vi "qCOV.vi"(0 "System no.":i32=1 min=1 max=4 step=1, 2 "ID to query":string[](array[string]), 3 "All IDs?":bool, 5 "error in":errorcluster) -> (14 "OL Velocity":dbl[](array[numeric]) format="%.6f", 19 "error out":errorcluster)   [LabVIEW 2020]
doc: "Returns current open loop velocity for specified IDs.\n\nE-870: Only one ID to query per command allowed."
panel:
  # "Returns current open loop velocity for specified IDs."
  # "Query"
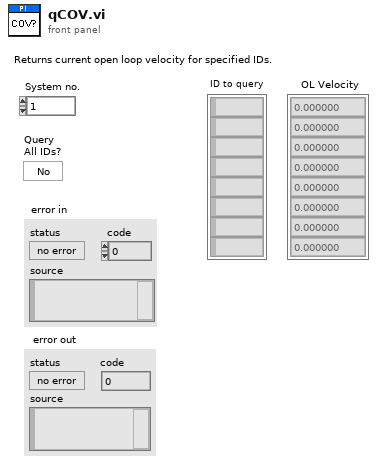
[diagram p1: front panel]
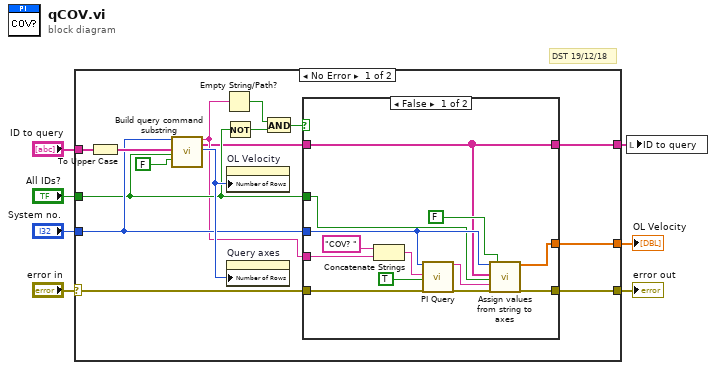
[diagram p0: block diagram]
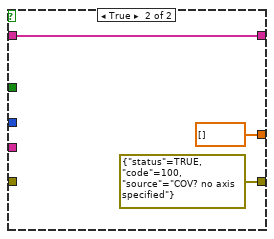
[diagram p2: hidden frame]
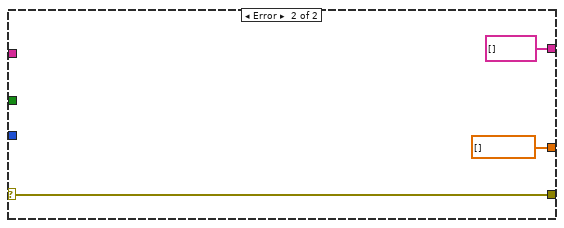
[diagram p3: hidden frame]
diagram:
  # "DST 19/12/18"
  n1 = case shown="No Error" "error in" {
    selector: "error in" -> [w11 w39]
    tunnel: [w22 dbl[] [] ("Values")] -> w7
    tunnel: "ID to query" -> [w21 _]
    tunnel: [w20 w39] -> w5
    tunnel: "System no." -> [w16 _]
    tunnel: [w8 string[] [] ("Axes to query out")] -> w3
    tunnel: "All IDs?" -> [w15 _]
    frame No Error {
      n2 = To Upper Case(1:w21) -> (0:w19:string[])
      n3 = call "Build query command substring.vi"("System no."=w16, "Axes to query in"=w19, "Query\nAll axes?"=w15, "For all axes: use\nAxis identifier?"=FALSE ("Axis identifier?")) -> ("Command substring"=w13:string, "Axes to query out"=w9:string[], "Number of rows"=w18:u32)  [unwired: 2 in, 11 out]
      n4 = Empty String/Path?(string/path=w13) -> (empty?=w12:bool)
      n5 = Not(x=w15) -> (.not. x?=w17:bool)
      n6 = property on="OL Velocity" class="Arr (strict)"("Number of Rows"=w18) -> ()  [unwired: 2 in, 2 out]
      n7 = property on="Query axes" class="Arr (strict)"("Number of Rows"=w18) -> ()  [unwired: 2 in, 2 out]
      n8 = And(x=w12, y=w17) -> (x .and. y?=w10:bool)
      n9 = case shown="False" w10 {
        tunnel: [w33 dbl[] [] ("Values")] -> w22
        tunnel: [w32 errorcluster {"status"=TRUE, "code"=100, "source"="COV? no axis specified"} ("error out")] -> w20
        tunnel: w9 -> [w23 w36]
        tunnel: w16 -> [w31 _]
        tunnel: w15 -> [w30 _]
        tunnel: w13 -> [w25 _]
        tunnel: w11 -> [w24 _]
        tunnel: [w23 w36] -> w8
        frame False {
          n10 = Concatenate Strings("COV? ", w25) -> (w34:string)
          n11 = call "PI Query.vi"("System no."=w31, "String to send"=w34, "Attach termination char.?"=TRUE ("Attach Linefeed?"), "error in"=w24) -> ("String read"=w27:string, "error out"=w26:errorcluster)  [unwired: 3 in, 11 out]
          n12 = call "Assign values from string to axes.vi"("System no."=w31, "Queried axes"=w23, "All axes queried?"=w30, "Input String"=w27, "error in"=w26, "Axes related?"=FALSE) -> ("Values"=w33:dbl[], "error out"=w32:errorcluster)  [unwired: 3 in, 9 out]
        }
        frame True {
        }
      }
    }
    frame Error {
    }
  }
  "error out" <- w5
  "OL Velocity" <- w7
  n13 = local write "ID to query"(w3) -> ()
